vi "Process Read Data.vi"(1 "Bytes Read Count":u64, 2 "Data In":u8[](array[numeric])) -> (0 "Data Out":u8[](array[numeric]))   [LabVIEW 2018, in "Toolkit.lvlib" / "Channel.lvclass"]
uses:
  Channel.lvclass
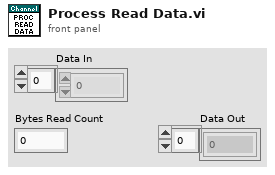
[diagram p1: front panel]
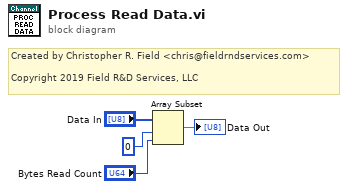
[diagram p0: block diagram]
diagram:
  # "Created by Christopher R. Field <chris@fieldrndservices.com>\n\nCopyright 2019 Field R&D Services, LLC"
  n1 = Array Subset(array="Data In", index=0, length="Bytes Read Count") -> (→"Data Out":u8[])
